vi "Pick & Place Status.vi"() -> ()   [LabVIEW 2021]
uses:
  Controls/Pick & Place.ctl
panel:
  in  "Pick & Place Status":T1
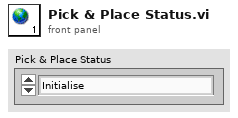
[diagram p1: front panel]
types:
  T1 = typedef "Pick & Place.ctl" = enum16{"Initialise", "Singling ON", "Front Vertical SOL", "Rear Vertical SOL", "ON Rotary", "Front Vertical SOL_2", "Bowler ON", "Rear Vertical SOL_2", "OFF Rotary", "Done", "Error"}
diagram:
